vi "read non-filtered apstream log.vi"() -> ()   [LabVIEW 2018]
panel:
  out "unsigned byte array":u8[](array[numeric]) format="%x"
  out "data":string
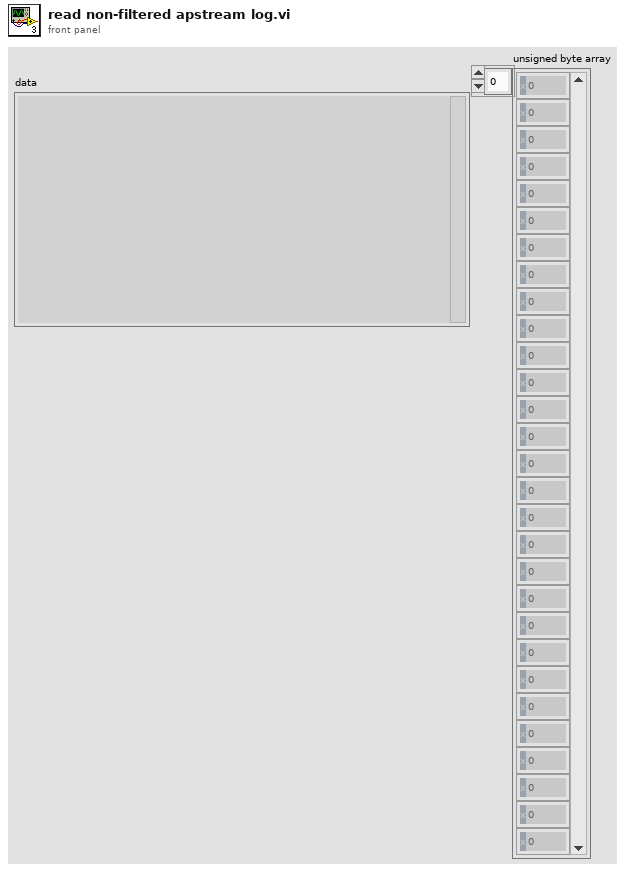
[diagram p1: front panel]
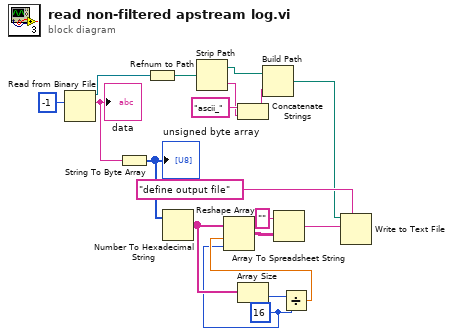
[diagram p0: block diagram]
diagram:
  w8 = 16 ("y")
  n1 = Read from Binary File(10:-1 ("count (1)")) -> (2:w17:string, 3:w7:refnum<file>)  [unwired: 5 in, 2 out]
  "data" <- w17
  n2 = String To Byte Array(string=w17) -> (unsigned byte array=w16:u8[])
  "unsigned byte array" <- w16
  n3 = Refnum to Path(1:w7) -> (0:w6:path)
  n4 = Number To Hexadecimal String(2:w16) -> (0:w10:string[])  [unwired: 1 in]
  n5 = Strip Path(path=w6) -> (stripped path=w5:path, name=w2:string)
  n6 = Concatenate Strings("ascii_" ("string"), w2) -> (w1:string)
  n7 = Array Size(array=w10) -> (size(s)=w14:i32)
  n8 = Build Path(base path=w5, name or relative path=w1) -> (appended path=w4:path)
  n9 = Divide(x=w14, y=w8) -> (x/y=w9:dbl)
  n10 = Reshape Array(w10, w9, w8) -> (w12:string[][])
  n11 = Array To Spreadsheet String(array=w12, 3:"" ("format string")) -> (spreadsheet string=w13:string)  [unwired: 1 in]
  n12 = Write to Text File(prompt (Choose or enter file path)="define output file", file (use dialog)=w4, text=w13) -> ()  [unwired: 1 in, 3 out]
